vi "Initialize.vi"(11 "Initialize in":refnum<class "Initialize.lvclass">) -> (0 "error out":errorcluster, 3 "Initialize out":refnum<class "Initialize.lvclass">)   [LabVIEW 2021, in "AAM.lvlib" / "Initialize.lvclass"]
uses:
  Initialize.lvclass
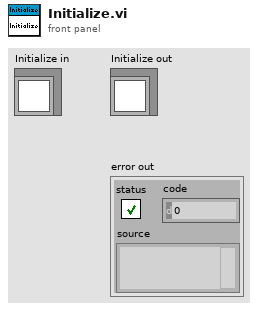
[diagram p1: front panel]
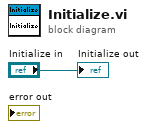
[diagram p0: block diagram]
diagram:
  "Initialize out" <- "Initialize in"
